vi "solar Private Data.vi"(8 "error in (no error)":errorcluster, 10 "Default LVClass":refnum<class "solar.lvclass">, 11 "solar in":refnum<class "solar.lvclass">) -> (0 "error out":errorcluster, 3 "solar out":refnum<class "solar.lvclass">)   [LabVIEW 2018, in "solar.lvclass"]
doc: "Override this function set the LabVIEW class private data. This is used when a target class is loaded by name and custom references need to be initialized without accessors."
uses:
  solar.lvclass
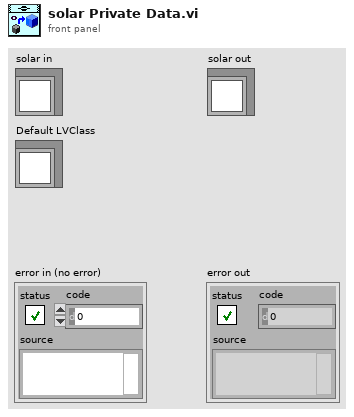
[diagram p1: front panel]
types:
  T1 = typedef "solar_ctl SOLAR Refnum.ctl" = refnum<k1>
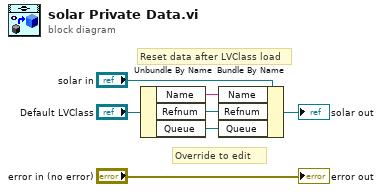
[diagram p0: block diagram]
diagram:
  # "Override to edit"
  # "Reset data after LVClass load"
  n1 = Unbundle By Name("Default LVClass") -> ("Name"=w6:string, "Refnum"=w5:T1, "Queue"=w4:refnum<queue>)
  n2 = Bundle By Name(cluster="solar in", "Name"=w6, "Refnum"=w5, "Queue"=w4) -> (→"solar out":refnum<class "solar.lvclass">)
  "error out" <- "error in (no error)"
